vi "Reply.vi"(4 "Is Priority":bool, 6 "Sender":refnum<class "Sender.lvclass">, 7 "Actor in":refnum<class "Actor.lvclass">) -> (0 "Error out":errorcluster)   [LabVIEW 2025, in "jettl.lvlib" / "Destroy Msg.lvlib"]
uses:
  Destroy Msg.lvlib
  Destroy Msg/Destroy Msg.lvclass
  C:/git/jettl/src/jettl/jettl/Destroy Msg/Destroy Msg/Destroy Msg.lvclass
  C:/git/jettl/src/jettl/jettl/Msg/Msg.lvclass
  Actor/Actor/Actor.lvclass
  Sender/Sender/Sender.lvclass
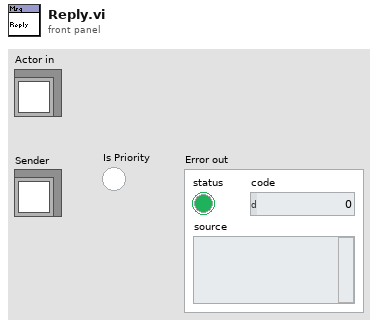
[diagram p1: front panel]
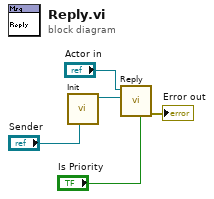
[diagram p0: block diagram]
diagram:
  n1 = call "Init.vi"("Sender"="Sender") -> ("Destroy Msg out"=w1:refnum<class "Destroy Msg.lvclass">)  [unwired: 10 in]
  n2 = call-dynamic "Reply.vi"("Is Priority"="Is Priority", "Msg"=w1, "Actor in"="Actor in") -> ("Error out"=→"Error out":errorcluster)  [unwired: 8 in]
